vi "TCP Daemon.vi"(8 "UUID":string, 9 "data model":refnum<class "Device Data Model.lvclass">, 10 "transmission data unit":refnum<class "Transmission Data Unit.lvclass">, 11 "TCP slave in":refnum<class "TCP Slave.lvclass">) -> ()   [LabVIEW 2020, in "SubVIs.lvlib" / "TCP Slave.lvclass"]
doc: "This daemon waits for new connections and launches connection handlers as needed. It also obtains a local reference to the quit notification, and waits for that to occur."
uses:
  <vilib>/Modbus/subvis/Protocol/TCP/TCP Slave/TCP Slave.lvclass
  <vilib>/Modbus/subvis/Transmission Data Unit (ADU)/Transmission Data Unit/Transmission Data Unit.lvclass
  C:/builds/penguin/iak/lvdsc/trunk/20.0/lv/vi.lib/Modbus/subvis/Protocol/Interfaces/Network Slave/Network Slave.lvclass
  <vilib>/Modbus/subvis/Data and Functions/Device Data Model/Device Data Model.lvclass
  <vilib>/Modbus/subvis/Protocol/Interfaces/Network Slave/Network Slave.lvclass/Network Slave.ctl
  <vilib>/Modbus/subvis/Protocol/TCP/TCP Slave/TCP Slave.lvclass/TCP Slave.ctl
  <vilib>/Modbus/subvis/Protocol/TCP/TCP Slave/Remove Unused Connections.vi
  <vilib>/Modbus/subvis/Protocol/TCP/TCP Slave/Remove Connection Record Reference.vi
  <vilib>/Modbus/subvis/Protocol/Interfaces/Network Slave/Network Slave.lvclass
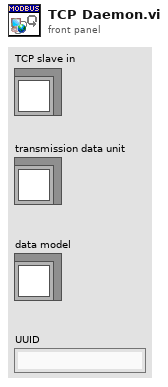
[diagram p1: front panel]
types:
  T1 = enum16{"Check Notifier", "Check for Available Connection Slot", "Wait on Connection", "Quit"}
  T2 = enum16{"Not Started", "Running", "Error", "Stopped"}
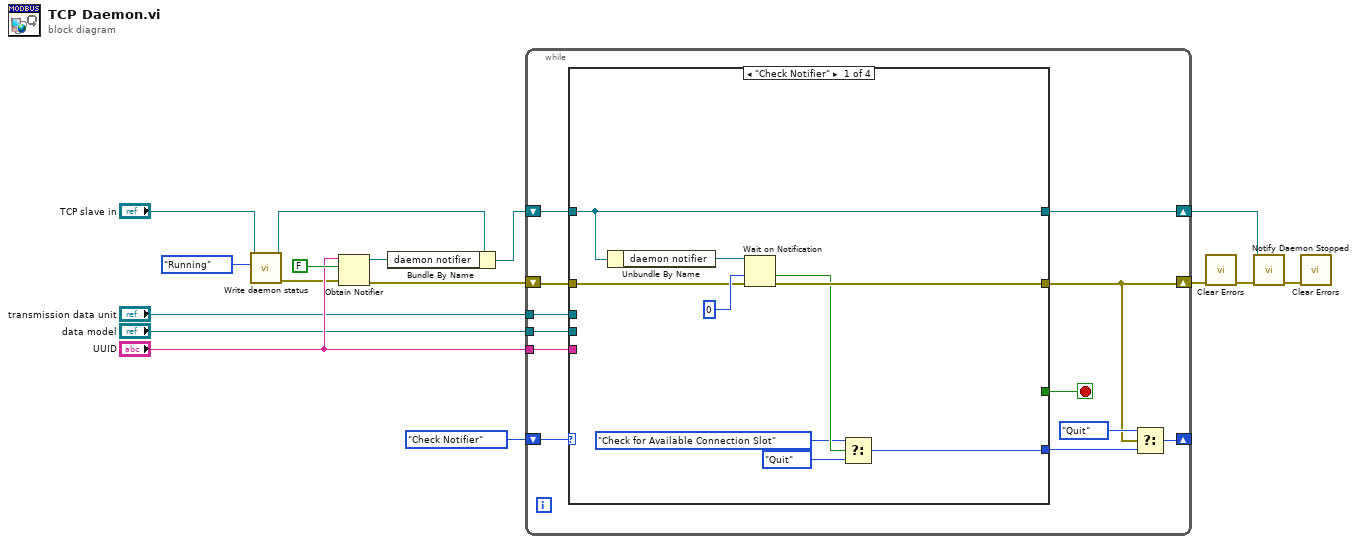
[diagram p0: block diagram]
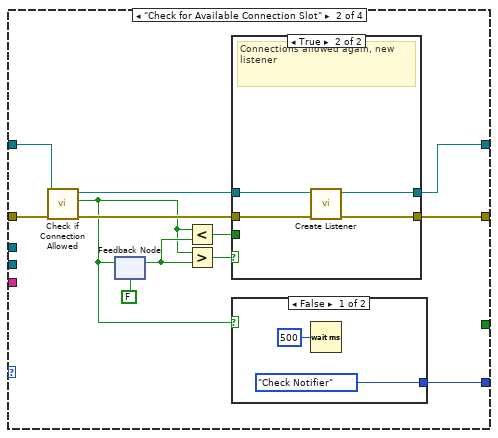
[diagram p2: hidden frame]
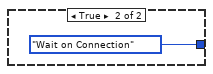
[diagram p3: hidden frame]
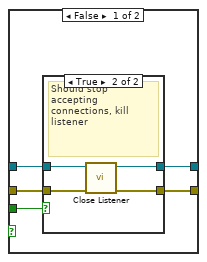
[diagram p4: hidden frame]
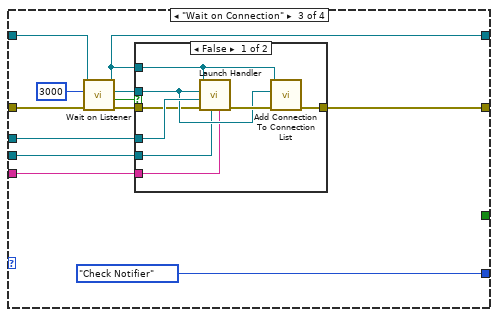
[diagram p6: hidden frame]
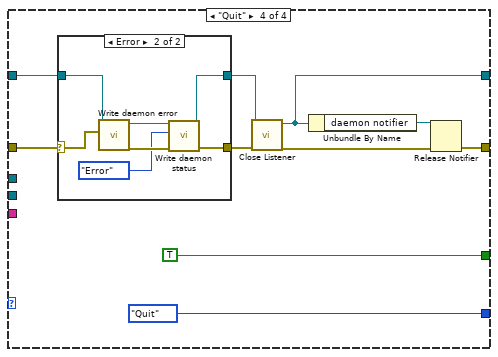
[diagram p8: hidden frame]
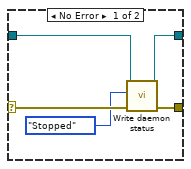
[diagram p9: hidden frame]
diagram:
  n1 = call <vilib>:"Write daemon status.vi"("daemon status"=T2."Running", "network slave in"="TCP slave in") -> ("error out"=w6:errorcluster, "network slave out"=w8:refnum<class "TCP Slave.lvclass">)  [unwired: 8 in]
  n2 = Obtain Notifier(name (unnamed)="UUID", notification data type=FALSE, error in (no error)=w6) -> (notifier out=w14:refnum<notifier>, error out=w9:errorcluster)  [unwired: 1 in, 1 out]
  n3 = Bundle By Name(cluster=w8, "daemon notifier"=w14) -> (w13:refnum<class "TCP Slave.lvclass">)
  n4 = while {
    shift-right: [w26] -> _
    shift-left: T1."Check Notifier" -> [w28]
    tunnel: "UUID" -> [w23]
    tunnel: "data model" -> [w22]
    tunnel: "transmission data unit" -> [w21]
    shift-right: [w20] -> w2
    shift-left: w9 -> [w19]
    shift-right: [w17] -> w4
    shift-left: w13 -> [w27]
    stop <- w18 stop-if-true
    n5 = case shown="\"Check Notifier\"" w28 {
      tunnel: w27 -> [w29 w48 w78 w97]
      tunnel: [w36 w42 w68 w94] -> w20
      tunnel: [w31 w38 T1."Check Notifier" T1."Quit"] -> w24
      tunnel: w23 -> [_ _ w75 _]
      tunnel: w22 -> [_ _ w74 _]
      tunnel: w21 -> [_ _ w73 _]
      tunnel: w19 -> [w30 w49 w72 w98]
      tunnel: [_ _ _ TRUE] -> w18
      tunnel: [w29 w43 w71 w89] -> w17
      frame "Check Notifier" {
        n6 = Unbundle By Name(w29) -> ("daemon notifier"=w37:refnum<notifier>)
        n7 = Wait on Notification(notifier=w37, timeout in ms (-1)=0, error in (no error)=w30) -> (timed out?=w35:bool, error out=w36:errorcluster)  [unwired: 1 in, 2 out]
        n8 = Select(t=T1."Check for Available Connection Slot", s=w35, f=T1."Quit") -> (s? t:f=w31:T1)
      }
      frame "Check for Available Connection Slot" {
        n9 = call <vilib>:"Check if Connection Allowed.vi"("error in (no error)"=w49, "TCP slave in"=w48) -> ("error out"=w45:errorcluster, "connection allowed"=w39:bool, "TCP slave out"=w44:refnum<class "TCP Slave.lvclass">)  [unwired: 7 in]
        n10 = feedback-in #1(w39) -> ()
        n11 = feedback #1(FALSE) -> (w41:bool)
        n12 = Less?(x=w39, y=w41) -> (x < y?=w40:bool)
        n13 = Greater?(x=w39, y=w41) -> (0:w46:bool)
        n14 = case shown="True" w46 {
          tunnel: w45 -> [w55 w66]
          tunnel: w44 -> [w56 w67]
          tunnel: [w53 w65] -> w43
          tunnel: [w54 w64] -> w42
          tunnel: w40 -> [w57 _]
          frame False {
            n15 = case shown="True" w57 {
              tunnel: w56 -> [w59 w63]
              tunnel: w55 -> [w58 w62]
              tunnel: [w58 w61] -> w54
              tunnel: [w59 w60] -> w53
              frame False {
              }
              frame True {
                # "Should stop accepting connections, kill listener"
                n16 = call <vilib>:"Close Listener.vi"("error in (no error)"=w62, "TCP slave in"=w63) -> ("error out"=w61:errorcluster, "TCP slave out"=w60:refnum<class "TCP Slave.lvclass">)  [unwired: 8 in]
              }
            }
          }
          frame True {
            # "Connections allowed again, new listener"
            n17 = call <vilib>:"Create Listener.vi"("error in (no error)"=w66, "TCP slave in"=w67) -> ("error out"=w64:errorcluster, "TCP slave out"=w65:refnum<class "TCP Slave.lvclass">)  [unwired: 8 in]
          }
        }
        n18 = case shown="False" w39 {
          tunnel: [T1."Check Notifier" T1."Wait on Connection"] -> w38
          frame False {
            n19 = Wait (ms)(milliseconds to wait=u32 500) -> ()  [unwired: 1 out]
          }
          frame True {
          }
        }
      }
      frame "Wait on Connection" {
        n20 = call-dynamic "Wait on Listener.vi"("error in (no error)"=w72, "timeout ms (wait forever: -1)"=3000, "TCP slave in"=w78) -> ("error out"=w69:errorcluster, "timed out?"=w70:bool, "connection reference"=w76:refnum<data-value>, "TCP slave out"=w71:refnum<class "TCP Slave.lvclass">)  [unwired: 5 in]
        n21 = case shown="False" w70 {
          tunnel: w76 -> [w84 _]
          tunnel: w71 -> [w83 _]
          tunnel: w75 -> [w82 _]
          tunnel: w74 -> [w81 _]
          tunnel: w73 -> [w87 _]
          tunnel: [w86 w88] -> w68
          tunnel: w69 -> [w80 w88]
          frame False {
            n22 = call <vilib>:"Launch Handler.vi"("UUID"=w82, "data model"=w81, "error in (no error)"=w80, "transmission data unit"=w87, "connection reference"=w84, "TCP slave"=w83) -> ("error out"=w85:errorcluster)  [unwired: 5 in]
            n23 = call <vilib>:"Add Connection To Connection List.vi"("error in (no error)"=w85, "data value reference"=w84, "TCP slave in"=w83) -> ("error out"=w86:errorcluster)  [unwired: 8 in]
          }
          frame True {
          }
        }
      }
      frame "Quit" {
        n24 = case shown="Error" w98 {
          selector: w98 -> [w100 w105]
          tunnel: [w101 w107] -> w96
          tunnel: w97 -> [w103 w110]
          tunnel: [w102 w108] -> w95
          frame No Error {
            n25 = call <vilib>:"Write daemon status.vi"("error in (no error)"=w100, "daemon status"=T2."Stopped", "network slave in"=w103) -> ("error out"=w101:errorcluster, "network slave out"=w102:refnum<class "TCP Slave.lvclass">)  [unwired: 7 in]
          }
          frame Error {
            n26 = call <vilib>:"Write daemon error.vi"("daemon error"=w105, "network slave in"=w110) -> ("error out"=w106:errorcluster, "network slave out"=w109:refnum<class "TCP Slave.lvclass">)  [unwired: 8 in]
            n27 = call <vilib>:"Write daemon status.vi"("error in (no error)"=w106, "daemon status"=T2."Error", "network slave in"=w109) -> ("error out"=w107:errorcluster, "network slave out"=w108:refnum<class "TCP Slave.lvclass">)  [unwired: 7 in]
          }
        }
        n28 = call <vilib>:"Close Listener.vi"("error in (no error)"=w96, "TCP slave in"=w95) -> ("error out"=w90:errorcluster, "TCP slave out"=w89:refnum<class "TCP Slave.lvclass">)  [unwired: 8 in]
        n29 = Unbundle By Name(w89) -> ("daemon notifier"=w91:refnum<notifier>)
        n30 = Release Notifier(notifier=w91, error in (no error)=w90) -> (error out=w94:errorcluster)  [unwired: 1 in, 2 out]
      }
    }
    n31 = Select(t=T1."Quit", s=w20, f=w24) -> (s? t:f=w26:T1)
  }
  n32 = call <vilib>:"Clear Errors.vi"("error in (no error)"=w2) -> ("error out"=w3:errorcluster)  [unwired: 5 in, 1 out]
  n33 = call <vilib>:"Notify Daemon Stopped.vi"("error in (no error)"=w3, "Network Slave in"=w4) -> ("error out"=w1:errorcluster)  [unwired: 8 in, 1 out]
  n34 = call <vilib>:"Clear Errors.vi"("error in (no error)"=w1) -> ()  [unwired: 5 in, 2 out]
